vi "Initialize.vi"(8 "error in (no error)":errorcluster) -> (0 "error out":errorcluster, 3 "Engine out":refnum<class "Engine.lvclass">)   [LabVIEW 2019, in "RT_Game.lvlib" / "Engine.lvclass"]
uses:
  Engine.lvclass
  MainMenu/MainMenu.lvclass
  C:/Users/FreshBob/Dropbox/VIs/myRIO_GameConsole/RT/RT_Game/Game/Game.lvclass
  Engine.lvclass/Engine.ctl
  <vilib>/FPGAPlugInAG/myRIO-1900/niLvFpga_Open_myRIO-1900.vi
  <vilib>/FPGAPlugInAG/myRIO-1900/niLvFpga_Download_myRIO-1900.vi
  <vilib>/FPGAPlugInAG/myRIO-1900/niLvFpga_Run_myRIO-1900.vi
  <vilib>/rvi/interface/nirviOpenFPGA/nirviOpenFPGA.xnode
  FPGA_Interface.ctl
  FPGA Bitfiles/myriogameconsole_FPGATarget_Main_ntsPRcBZGxk.lvbitx
  <vilib>/rvi/interface/nirviMethod/nirviMethod.xnode
  Game/Game.lvclass
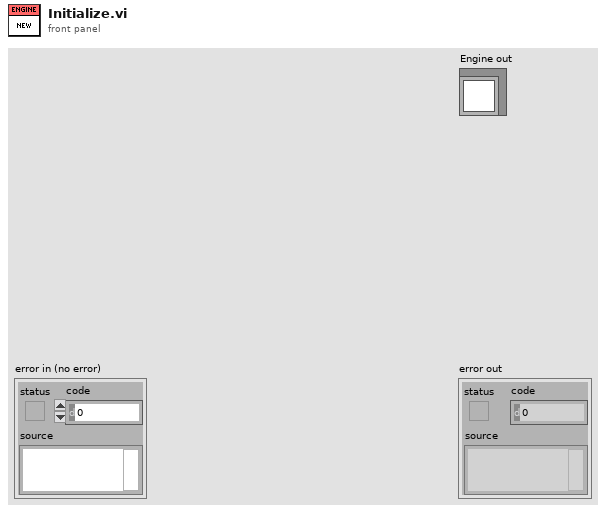
[diagram p1: front panel]
types:
  T1 = typedef "FPGA_Interface.ctl" = refnum<k20>
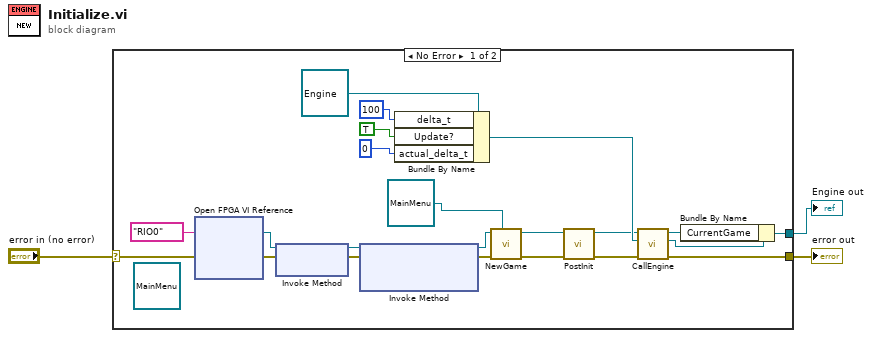
[diagram p0: block diagram]
diagram:
  n1 = case shown="No Error" "error in (no error)" {
    selector: "error in (no error)" -> [w22 w26]
    tunnel: [w12 w26] -> w2
    tunnel: [w9 _] -> w1
    frame No Error {
      (unwired) refnum<class "MainMenu.lvclass"> refnum ("RT_Game.lvlib:MainMenu.lvclass")
      n2 = xnode "Open FPGA VI Reference"("error in"=w22, "resource name"=tag "RIO0") -> ("FPGA VI Reference Out"=w16:T1, "error out"=w23:errorcluster)
      n3 = xnode "Invoke Method"("FPGA VI Reference In"=w16, "error in"=w23) -> ("FPGA VI Reference Out"=w14:T1, "error out"=w17:errorcluster)
      n4 = xnode "Invoke Method"("FPGA VI Reference In"=w14, "error in"=w17) -> ("FPGA VI Reference Out"=w13:T1, "error out"=w15:errorcluster)  [unwired: 1 in]
      n5 = Bundle By Name(cluster=refnum<class "Engine.lvclass"> refnum ("Engine out"), "delta_t"=u16 100, "Update?"=TRUE, "actual_delta_t"=u16 0) -> (w11:refnum<class "Engine.lvclass">)
      n6 = call-dynamic "NewGame.vi"("GameType (ChildObject)"=refnum<class "MainMenu.lvclass"> refnum ("RT_Game.lvlib:MainMenu.lvclass"), "error in (no error)"=w15, "FPGA_ref"=w13) -> ("error out"=w21:errorcluster, "Game out"=w6:refnum<class "MainMenu.lvclass">)  [unwired: 7 in]
      n7 = call "PostInit.vi"("error in (no error)"=w21, "Game in"=w6) -> ("error out"=w7:errorcluster, "Game out"=w5:refnum<class "MainMenu.lvclass">)  [unwired: 8 in]
      n8 = call-dynamic "CallEngine.vi"("error in (no error)"=w7, "RT_Game.lvlib:Engine.lvclass"=w11, "MainMenu in"=w5) -> ("error out"=w12:errorcluster, "RT_Game.lvlib:Engine.lvclass 2"=w10:refnum<class "Engine.lvclass">, "MainMenu out"=w8:refnum<class "MainMenu.lvclass">)  [unwired: 6 in]
      n9 = Bundle By Name(cluster=w10, "CurrentGame"=w8) -> (w9:refnum<class "Engine.lvclass">)
    }
    frame Error {
    }
  }
  "error out" <- w2
  "Engine out" <- w1
